vi "Player Info.vi"(11 "DNatt in":refnum<class "DNatt.lvclass">) -> (0 "Defeat Speech":string, 1 "Victory Speech":string, 2 "Name":string, 3 "DNatt out":refnum<class "DNatt.lvclass">)   [LabVIEW 2015, in "DNatt.lvclass"]
uses:
  DNatt.lvclass
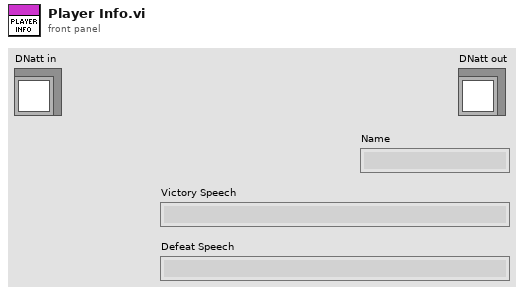
[diagram p1: front panel]
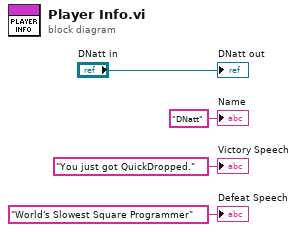
[diagram p0: block diagram]
diagram:
  "DNatt out" <- "DNatt in"
  "Name" <- "DNatt" ("Name")
  "Victory Speech" <- "You just got QuickDropped." ("Victory Speech")
  "Defeat Speech" <- "World's Slowest Square Programmer" ("Defeat Speech")
